vi "PRAT Seperate Data.vi"(8 "Error In":errorcluster, 10 "PRAT Power Data":string[][](array[string])=[["Power (Watts) - Station A", "1"], ["Power (Watts) - Station B", "2"], ["Power (Watts) - Station C", "3"], ["Power (Watts) - Station D", "4"], ["WattHours (Wh) - Station A", "5"], ["WattHours (Wh) - Station B", "6"], ["WattHours (Wh) - Station C", "7"], ["WattHours (Wh) - Station D", "8"]], 11 "Prat Station":string="Station D") -> (0 "Error Out":errorcluster, 2 "RMS Current (Amps)":dbl, 3 "Station Power Data":string[][](array[string])=[["Power (Watts) - Station D", "4"], ["WattHours (Wh) - Station D", "8"]])   [LabVIEW 2016]
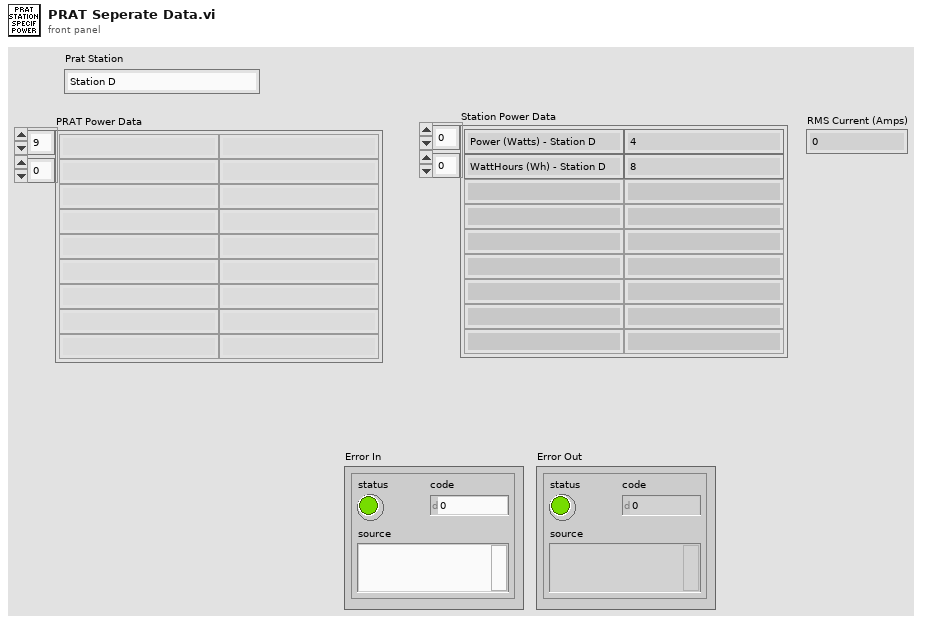
[diagram p1: front panel]
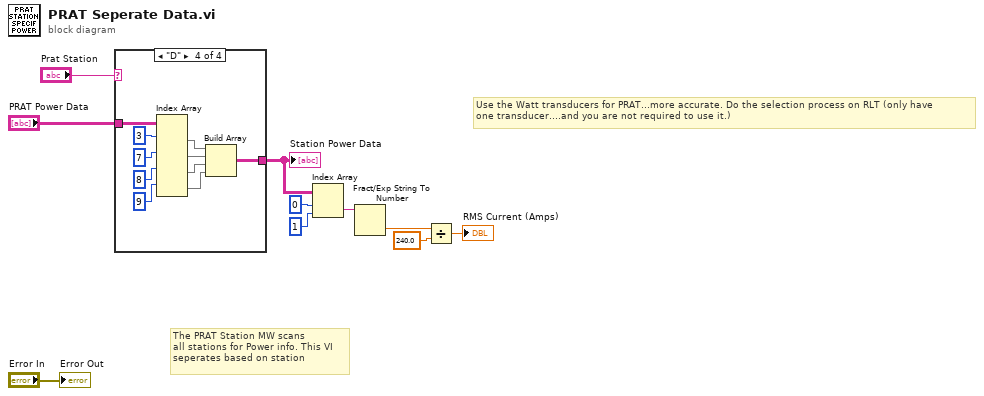
[diagram p0: block diagram]
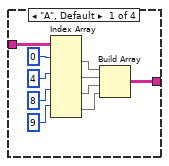
[diagram p2: hidden frame]
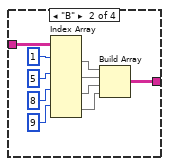
[diagram p3: hidden frame]
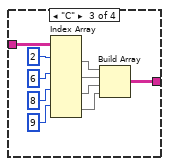
[diagram p4: hidden frame]
diagram:
  # "Use the Watt transducers for PRAT...more accurate. Do the selection process on RLT (only have\none transducer....and you are not required to use it.)"
  # "The PRAT Station MW scans\nall stations for Power info. This VI\nseperates based on station"
  n1 = case shown="\"D\"" "Prat Station" {
    tunnel: "PRAT Power Data" -> [w18 w28 w38 w48]
    tunnel: [w15 w25 w35 w45] -> w7
    frame "A", Default {
      n2 = Index Array(array=w18, index (row) #1=0 ("index (row)"), index (row) #2=4 ("index (row)"), index (row) #3=8 ("index (row)"), index (row) #4=9 ("index (row)")) -> (element #1=w17:string[], element #2=w16:string[], element #3=w13:string[], element #4=w11:string[])  [unwired: 4 in]
      n3 = Build Array(w17, w16, w13, w11) -> (w15:string[][])
    }
    frame "B" {
      n4 = Index Array(array=w28, index (row) #1=1 ("index (row)"), index (row) #2=5 ("index (row)"), index (row) #3=8 ("index (row)"), index (row) #4=9 ("index (row)")) -> (element #1=w27:string[], element #2=w26:string[], element #3=w23:string[], element #4=w21:string[])  [unwired: 4 in]
      n5 = Build Array(w27, w26, w23, w21) -> (w25:string[][])
    }
    frame "C" {
      n6 = Index Array(array=w38, index (row) #1=2 ("index (row)"), index (row) #2=6 ("index (row)"), index (row) #3=8 ("index (row)"), index (row) #4=9 ("index (row)")) -> (element #1=w37:string[], element #2=w36:string[], element #3=w33:string[], element #4=w31:string[])  [unwired: 4 in]
      n7 = Build Array(w37, w36, w33, w31) -> (w35:string[][])
    }
    frame "D" {
      n8 = Index Array(array=w48, index (row) #1=3 ("index (row)"), index (row) #2=7 ("index (row)"), index (row) #3=8 ("index (row)"), index (row) #4=9 ("index (row)")) -> (element #1=w47:string[], element #2=w46:string[], element #3=w43:string[], element #4=w41:string[])  [unwired: 4 in]
      n9 = Build Array(w47, w46, w43, w41) -> (w45:string[][])
    }
  }
  "Station Power Data" <- w7
  n10 = Index Array(array=w7, index (row)=0, index (col)=1 ("disabled index (col)")) -> (element=w4:string)
  n11 = Fract/Exp String To Number(string=w4) -> (number=w2:dbl)  [unwired: 3 in, 1 out]
  n12 = Divide(x=w2, y=240.0) -> (x/y=→"RMS Current (Amps)":dbl)
  "Error Out" <- "Error In"
